vi "Build Async Wrapper.vi"(8 "error in (no error)":errorcluster, 11 "setup in":variant) -> (0 "error out":errorcluster, 3 "generated files":variant)   [LabVIEW 2020]
doc: "Wrapper for programatic build. This is intended to be called asynchronously."
uses:
  <vilib>/AppBuilder/AB_API_Simple/NI_App_Builder_API.lvlib
  <vilib>/AppBuilder/AB_API_Simple/Build (path).vi
  Build Setup.ctl
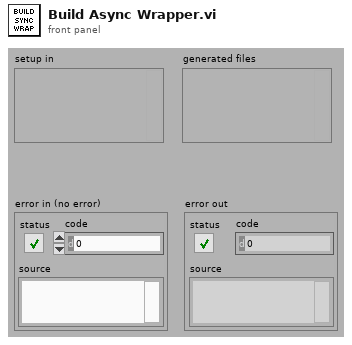
[diagram p1: front panel]
types:
  T1 = typedef "Build Setup.ctl" = cluster{"project path":path, "build spec name":string, "target name":string}
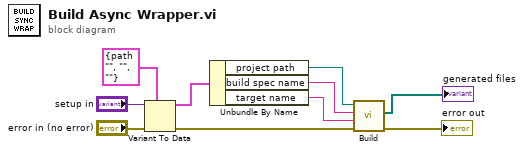
[diagram p0: block diagram]
diagram:
  n1 = Variant To Data(error in="error in (no error)", type=T1 {"project path"=path "", "build spec name"="", "target name"=""} ("build setup"), Variant="setup in") -> (data=w5:T1, error out=w6:errorcluster)
  n2 = Unbundle By Name(w5) -> ("project path"=w4:path, "build spec name"=w3:string, "target name"=w2:string)
  n3 = call-poly <vilib>:"Build.vi"("error in (no error)"=w6, "Name of target (My Computer)"=w2, "Name of build specification (if empty: build all)"=w3, "Path to project"=w4) -> ("error out"=→"error out":errorcluster, "Generated files"=→"generated files":path[])  [unwired: 6 in]
